vi "ReadConfigIniCluster.vi"(0 "更随产品型号变更？":bool, 1 "ConfigFlieName":string="DAQSetting.ini收参数.ini", 2 "ConfigOut":variant, 3 "ProductName":string="产品名称XXX", 5 "error in (no error)":errorcluster caption="错误输入（无错误）") -> (16 "ConfigOut":variant, 19 "error out":errorcluster caption="错误输出")   [LabVIEW 2020]
uses:
  <vilib>/Utility/config.llb/NI_LVConfig.lvlib
  DAQ_Base.lvclass
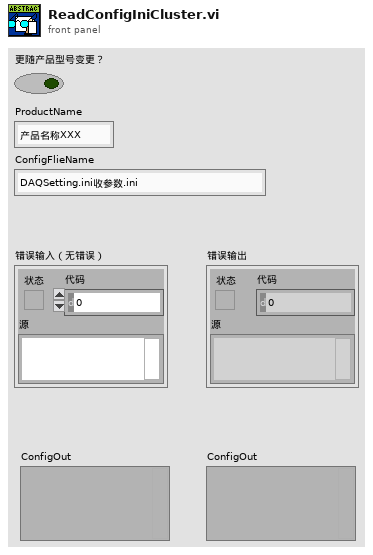
[diagram p1: front panel]
types:
  T1 = typedef "NI_LVConfig.lvlib/Config Data RefNum.ctl" = refnum<k1>
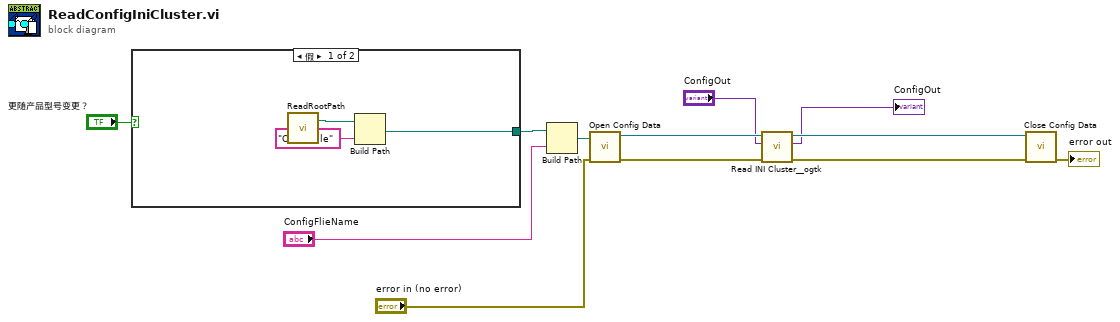
[diagram p0: block diagram]
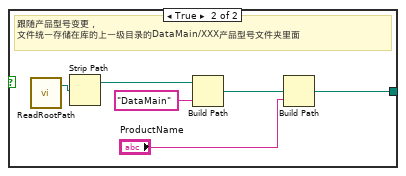
[diagram p2: hidden frame]
diagram:
  n1 = case shown="假" "更随产品型号变更？" {
    tunnel: [w13 w17] -> w9
    frame False {
      n2 = call "ReadRootPath.vi"() -> ("Root path"=w14:path)  [unwired: 19 in]
      n3 = Build Path(base path=w14, name or relative path="ConfigFile" ("ConfigFlieFolderName")) -> (appended path=w13:path)
    }
    frame True {
      # "跟随产品型号变更，\n文件统一存储在库的上一级目录的DataMain/XXX产品型号文件夹里面"
      n4 = call "ReadRootPath.vi"() -> ("Root path"=w19:path)  [unwired: 19 in]
      n5 = Strip Path(path=w19) -> (stripped path=w20:path)  [unwired: 1 out]
      n6 = Build Path(base path=w20, name or relative path="DataMain" ("ConfigFlieFolderName")) -> (appended path=w18:path)
      n7 = Build Path(base path=w18, name or relative path="ProductName") -> (appended path=w17:path)
    }
  }
  n8 = Build Path(base path=w9, name or relative path="ConfigFlieName") -> (appended path=w8:path)
  n9 = call <vilib>:"Open Config Data.vi"("error in (no error)"="error in (no error)", "configuration file path"=w8) -> ("error out"=w5:errorcluster, "refnum"=w4:T1)  [unwired: 7 in, 1 out]
  n10 = call <userlib>:"Read INI Cluster__ogtk.vi"("error in (no error)"=w5, "INI Fomatted Cluster Type"="ConfigOut", "refnum"=w4) -> ("error out"=w11:errorcluster, "INI Fomatted Cluster"=→"ConfigOut":variant, "dup refnum"=w12:T1)  [unwired: 4 in, 2 out]
  n11 = call <vilib>:"Close Config Data.vi"("error in (no error)"=w11, "refnum"=w12) -> ("error out"=→"error out":errorcluster)  [unwired: 8 in, 1 out]
